vi "Request UI Display (Cloneable)--template.vi"(6 "wait for reply (T)":bool=TRUE, 8 "error in (no error)":errorcluster, 10 "Scenario":T1, 11 "Module ID":i32=-1) -> (0 "error out":errorcluster, 3 "Accept?":bool)   [LabVIEW 2022 SP3, in "hse-dqmh-dynamicrequesters.lvlib"]
doc: "____\nHAMPEL SOFTWARE ENGINEERING v3.8.0 (2023-12-18 14:41)"
uses:
  hse-dqmh-dynamicrequesters.lvlib
  Controls/Module Display Scenarios.ctl
  hse-dqmh.lvlib
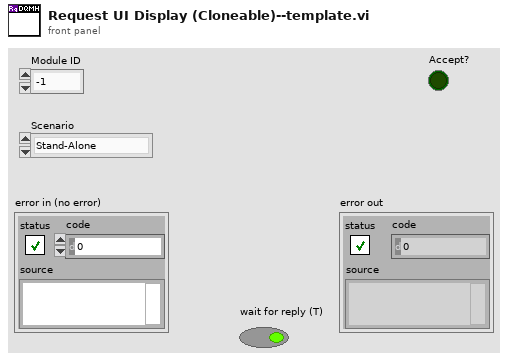
[diagram p1: front panel]
types:
  T1 = typedef "hse-dqmh.lvlib/Module Display Scenarios.ctl" = enum16{"Stand-Alone", "Managed"}
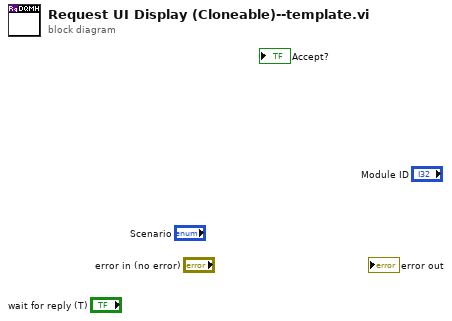
[diagram p0: block diagram]
diagram:
